vi "Load Profile.vi"(0 "Temp Chamber in":refnum<class "Temp Chamber.lvclass">, 5 "Profile Number":u32=1 min=1 step=1, 7 "Profile Name":string, 9 "Profile":string[][](array[string]), 11 "error in (no error)":errorcluster) -> (4 "Temp Chamber out":refnum<class "Temp Chamber.lvclass">, 15 "error out":errorcluster)   [LabVIEW 2018, in "Temp Chamber.lvlib" / "Temp Chamber.lvclass"]
doc: "This Override is used to load a Profile to the Temp Chamber. It requires a Profile Number and the profile information is passed as a 2D atring array."
uses:
  Temp Chamber.lvclass
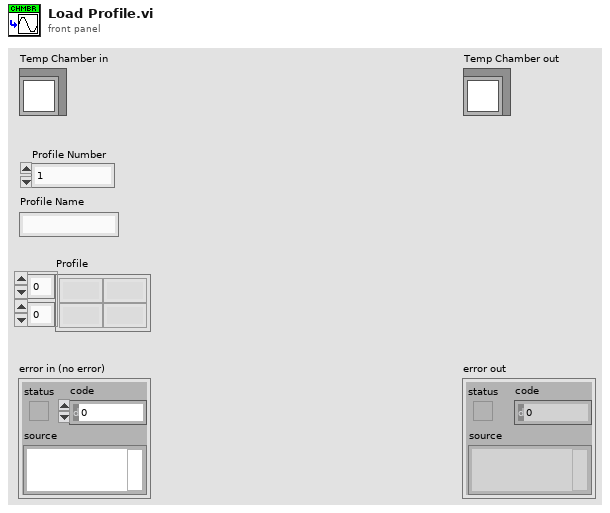
[diagram p1: front panel]
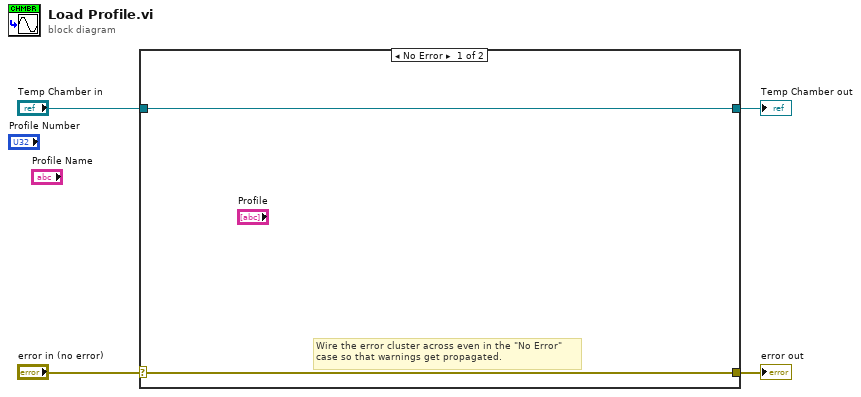
[diagram p0: block diagram]
diagram:
  n1 = case shown="No Error" "error in (no error)" {
    selector: "error in (no error)" -> [w5 w8]
    tunnel: [w5 w8] -> w3
    tunnel: [w6 w7] -> w1
    tunnel: "Temp Chamber in" -> [w6 w7]
    frame No Error {
      # "Wire the error cluster across even in the \"No Error\"\ncase so that warnings get propagated."
    }
    frame Error {
    }
  }
  "error out" <- w3
  "Temp Chamber out" <- w1
